vi "Order Properties from Dialog.vi"(10 "Original Properties":T1(array[cluster])=[{"Label"="a", "Tag"="a", "Property Type"=enum."Base", "Indent"=0, "Can Read?"=TRUE, "Can Write?"=TRUE, "Is Read?"=FALSE, "Is Write?"=TRUE, "Inactive Parent?"=FALSE, "Unwired?"=FALSE}, {"Label"="b", "Tag"="b", "Property Type"=enum."Scripting", "Indent"=0, "Can Read?"=TRUE, "Can Write?"=FALSE, "Is Read?"=FALSE, "Is Write?"=FALSE, "Inactive Parent?"=FALSE, "Unwired?"=FALSE}, {"Label"="c", "Tag"="c", "Property Type"=enum."Base", "Indent"=0, "Can Read?"=TRUE, "Can Write?"=TRUE, "Is Read?"=FALSE, "Is Write?"=FALSE, "Inactive Parent?"=FALSE, "Unwired?"=FALSE}, {"Label"="d", "Tag"="d", "Property Type"=enum."Private", "Indent"=0, "Can Read?"=TRUE, "Can Write?"=FALSE, "Is Read?"=FALSE, "Is Write?"=FALSE, "Inactive Parent?"=FALSE, "Unwired?"=FALSE}, {"Label"="E", "Tag"="E", "Property Type"=enum."Base", "Indent"=0, "Can Read?"=TRUE, "Can Write?"=TRUE, "Is Read?"=FALSE, "Is Write?"=TRUE, "Inactive Parent?"=FALSE, "Unwired?"=FALSE}, {"Label"="f", "Tag"="f", "Property Type"=enum."Base", "Indent"=0, "Can Read?"=TRUE, "Can Write?"=FALSE, "Is Read?"=FALSE, "Is Write?"=FALSE, "Inactive Parent?"=FALSE, "Unwired?"=FALSE}], 11 "Property Array In":T2(array[cluster])) -> (3 "Property Array Out":T2(array[cluster]))   [LabVIEW 2023]
doc: "Any repeated properties from dialog should be grouped and placed in Read then Write order.\n\nIf no change has happened to the dialog, the output array will be empty, so no actions occur after dialog closes."
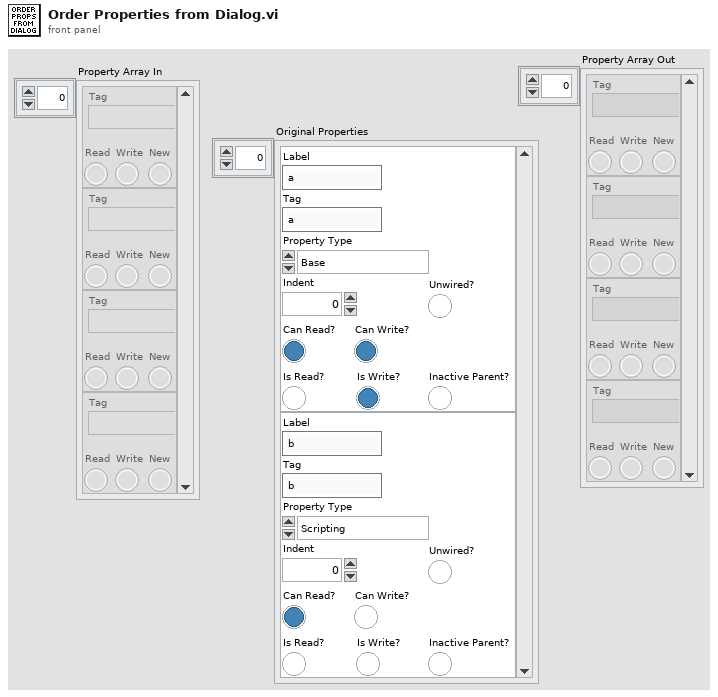
[diagram p1: front panel]
types:
  T1 = cluster{"Label":string, "Tag":string, "Property Type":enum16{"Unknown", "Base", "Scripting", "Private", "Deprecated", "None", "Divider"}, "Indent":u16, "Can Read?":bool, "Can Write?":bool, "Is Read?":bool, "Is Write?":bool, "Inactive Parent?":bool, "Unwired?":bool}[]
  T2 = cluster{"Tag":string, "Read":bool, "Write":bool, "New":bool}[]
  T3 = cluster{"Tag":string, "Read":bool, "Write":bool, "New":bool}
  T4 = cluster{"Label":string, "Tag":string, "Property Type":enum16{"Unknown", "Base", "Scripting", "Private", "Deprecated", "None", "Divider"}, "Indent":u16, "Can Read?":bool, "Can Write?":bool, "Is Read?":bool, "Is Write?":bool, "Inactive Parent?":bool, "Unwired?":bool}
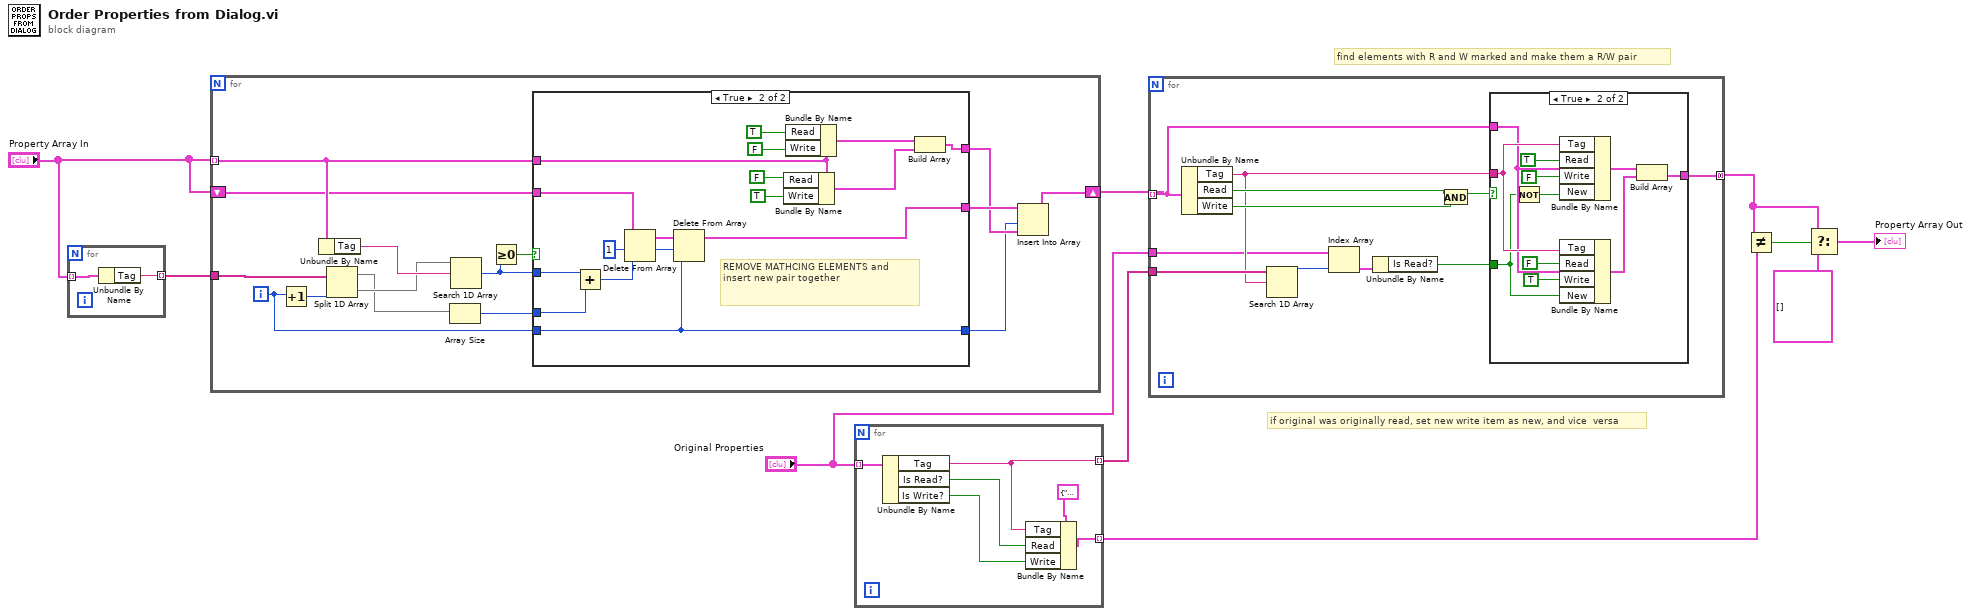
[diagram p0: block diagram]
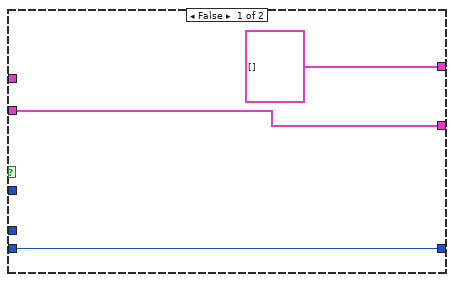
[diagram p2: hidden frame]
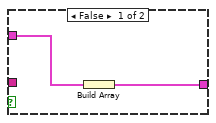
[diagram p3: hidden frame]
diagram:
  # "if original was originally read, set new write item as new, and vice  versa"
  # "find elements with R and W marked and make them a R/W pair"
  n1 = for {
    tunnel: "Property Array In" -> [w12] mode=indexing
    tunnel: [w11] -> w9 mode=indexing
    n2 = Unbundle By Name(w12) -> ("Tag"=w11:string)
  }
  n3 = for {
    tunnel: "Property Array In" -> [w25] mode=indexing
    shift-right: [w18] -> w8
    shift-left: "Property Array In" -> [w21]
    tunnel: w9 -> [w24]
    i -> [w14]
    n4 = Increment(x=w14) -> (x+1=w22:i32)
    n5 = Unbundle By Name(w25) -> ("Tag"=w26:string)
    n6 = Split 1D Array(array=w24, index=w22) -> (first subarray=w17:string[], second subarray=w23:string[])
    n7 = Array Size(array=w17) -> (size(s)=w16:i32)
    n8 = Search 1D Array(1D array=w23, element=w26) -> (index of element=w15:i32)  [unwired: 1 in]
    n9 = Greater Or Equal To 0?(x=w15) -> (x >= 0?=w27:bool)
    n10 = case shown="True" w27 {
      tunnel: w21 -> [w29 w46]
      tunnel: w25 -> [_ w38]
      tunnel: [T2 [] w40] -> w19
      tunnel: [w29 w31] -> w20
      tunnel: w16 -> [_ w36]
      tunnel: w15 -> [_ w33]
      tunnel: w14 -> [w28 w32]
      tunnel: [w28 w32] -> w13
      frame False {
      }
      frame True {
        w34 = 1 ("length")
        # "REMOVE MATHCING ELEMENTS and insert new pair together"
        n11 = Add(x=w33, y=w36) -> (x+y=w37:i32)
        n12 = Delete From Array(array=w46, length=w34, index=w37) -> (array with subset deleted=w35:T2)  [unwired: 1 out]
        n13 = Delete From Array(array=w35, length=w34, index=w32) -> (array with subset deleted=w31:T2)  [unwired: 1 out]
        n14 = Bundle By Name(cluster=w38, "Read"=FALSE, "Write"=TRUE) -> (w39:T3)
        n15 = Bundle By Name(cluster=w38, "Read"=TRUE, "Write"=FALSE) -> (w41:T3)
        n16 = Build Array(w41, w39) -> (w40:T2)
      }
    }
    n17 = Insert Into Array(array=w20, index=w13, new element=w19) -> (w18:T2)
  }
  n18 = for {
    tunnel: "Original Properties" -> [w52] mode=indexing
    tunnel: [w50] -> w7 mode=indexing
    tunnel: [w47] -> w5 mode=indexing
    n19 = Unbundle By Name(w52) -> ("Tag"=w50:string, "Is Read?"=w49:bool, "Is Write?"=w48:bool)
    n20 = Bundle By Name(cluster=T3 {"Tag"="", "Read"=FALSE, "Write"=FALSE, "New"=FALSE} ("Property Tree Element Value"), "Tag"=w50, "Read"=w49, "Write"=w48) -> (w47:T3)
  }
  n21 = for {
    tunnel: w8 -> [w60] mode=indexing
    tunnel: [w59] -> w3 mode=concatenating
    tunnel: w7 -> [w58]
    tunnel: "Original Properties" -> [w56]
    n22 = Unbundle By Name(w60) -> ("Tag"=w57:string, "Read"=w63:bool, "Write"=w62:bool)
    n23 = Search 1D Array(1D array=w58, element=w57) -> (index of element=w55:i32)  [unwired: 1 in]
    n24 = Index Array(array=w56, index=w55) -> (element=w54:T4)
    n25 = Unbundle By Name(w54) -> ("Is Read?"=w53:bool)
    n26 = And(x=w63, y=w62) -> (x .and. y?=w61:bool)
    n27 = case shown="True" w61 {
      tunnel: w57 -> [_ w72]
      tunnel: w60 -> [w65 w69]
      tunnel: [w64 w68] -> w59
      tunnel: w53 -> [_ w66]
      frame False {
        n28 = Build Array(w65) -> (w64:T2)
      }
      frame True {
        n29 = Not(x=w66) -> (.not. x?=w67:bool)
        n30 = Bundle By Name(cluster=w69, "Tag"=w72, "Read"=TRUE, "Write"=FALSE, "New"=w67) -> (w71:T3)
        n31 = Bundle By Name(cluster=w69, "Tag"=w72, "Read"=FALSE, "Write"=TRUE, "New"=w66) -> (w70:T3)
        n32 = Build Array(w71, w70) -> (w68:T2)
      }
    }
  }
  n33 = Not Equal?(x=w3, y=w5) -> (x != y?=w4:bool)
  n34 = Select(t=w3, s=w4, f=T2 []) -> (s? t:f=→"Property Array Out":T2)
